vi "test_intExpMA.vi"() -> ()   [LabVIEW 2016]
uses:
  <vilib>/rvi/DesktopExecutionNode/Execution/niFpgaDEN_Execute.vi
  <vilib>/rvi/DesktopExecutionNode/DesktopExecutionNode.xnode
panel:
  out "input":T1(array[cluster])
  out "output":T1(array[cluster])
  in  "ortInput":T2
  in  "expFactor":i8
  in  "numTicks":i32
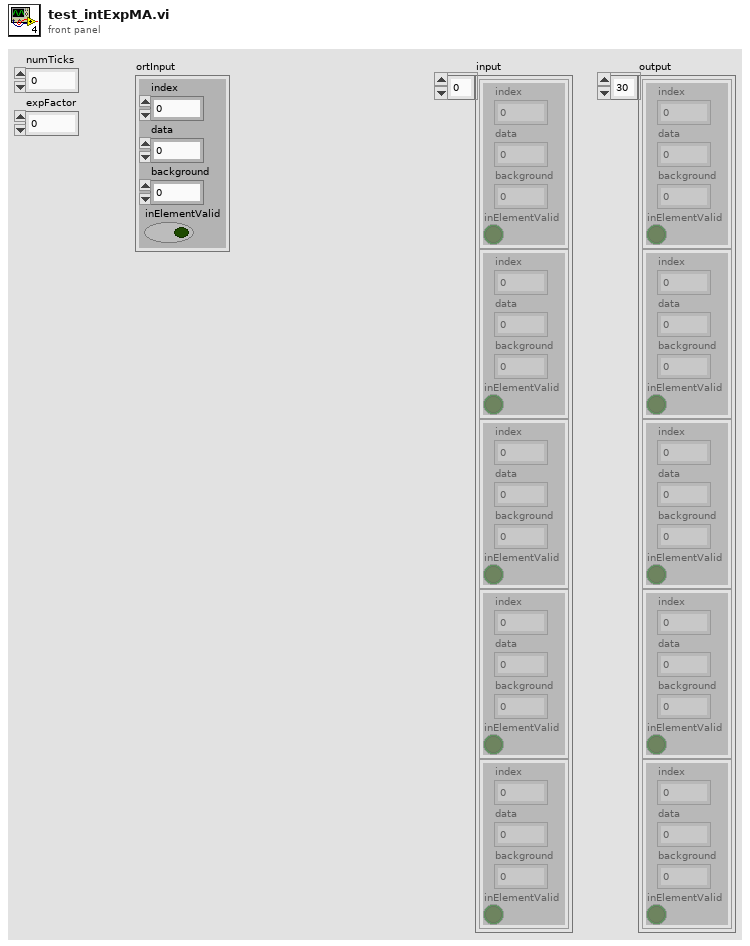
[diagram p1: front panel]
types:
  T1 = cluster{"index":u16, "data":i16, "background":i16, "inElementValid":bool}[]
  T2 = cluster{"index":u16, "data":i16, "background":i16, "inElementValid":bool}
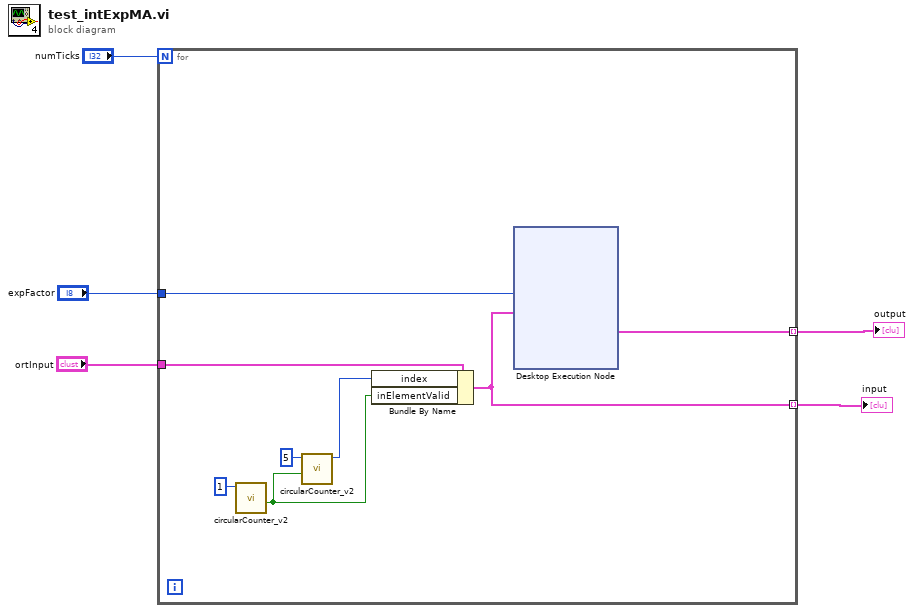
[diagram p0: block diagram]
diagram:
  n1 = for {
    N: "numTicks" -> [_]
    tunnel: "expFactor" -> [w13]
    tunnel: "ortInput" -> [w12]
    tunnel: [w11] -> w2 mode=indexing
    tunnel: [w7] -> w1 mode=indexing
    n2 = call "circularCounter_v2.vi"("maxCount"=u16 1) -> ("maxPulse"=w6:bool)  [unwired: 7 in, 3 out]
    n3 = call "circularCounter_v2.vi"("doStep"=w6, "maxCount"=u16 5) -> ("index"=w8:u16)  [unwired: 6 in, 3 out]
    n4 = Bundle By Name(cluster=w12, "index"=w8, "inElementValid"=w6) -> (w7:T2)
    n5 = xnode "Desktop Execution Node"("expFactor"=w13, "ortInput"=w7) -> ("ortOutput"=w11:T2)  [unwired: 1 in, 2 out]
  }
  "output" <- w2
  "input" <- w1
